vi "Initialize.vi"(8 "error in (no error)":errorcluster, 10 "Device":string) -> (0 "error out":errorcluster, 3 "Force Test Stand out":refnum<class "Force Test Stand.lvclass">)   [LabVIEW 2018, in "Force Test Stand.lvlib" / "Force Test Stand.lvclass"]
uses:
  Force Test Stand.lvclass
  Force Test Stand.lvclass/Force Test Stand.ctl
  builds/Configuration.lvlibp/Configuration.lvclass
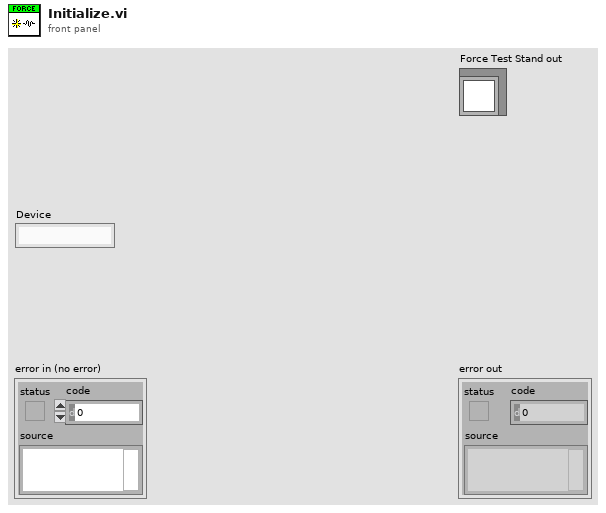
[diagram p1: front panel]
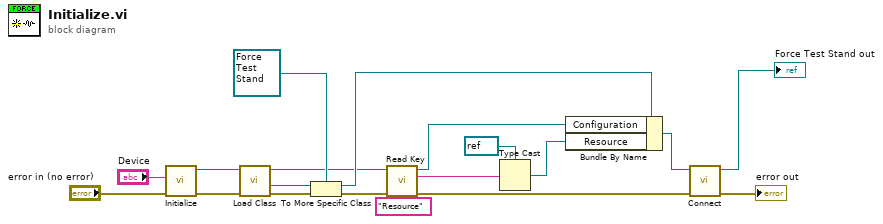
[diagram p0: block diagram]
diagram:
  n1 = call "Initialize.vi"("error in"="error in (no error)", "Device"="Device") -> ("error out"=w16:errorcluster, "Configuration out"=w17:refnum<class "Configuration.lvclass">)  [unwired: 8 in]
  n2 = call "Load Class.vi"("error in"=w16, "Configuration in"=w17) -> ("error out"=w15:errorcluster, "Class out"=w12:refnum<class>, "Configuration out"=w5:refnum<class "Configuration.lvclass">)  [unwired: 7 in]
  n3 = To More Specific Class(target class=refnum<class "Force Test Stand.lvclass"> refnum ("Force Test Stand.lvlib:Force Test Stand.lvclass"), reference=w12, error in=w15) -> (specific class reference=w13:refnum<class "Force Test Stand.lvclass">, error out=w11:errorcluster)
  n4 = call "Read Key.vi"("Key:"="Resource", "error in"=w11, "Configuration in"=w5) -> ("error out"=w10:errorcluster, "Value"=w6:string, "Configuration out"=w3:refnum<class "Configuration.lvclass">)  [unwired: 6 in]
  n5 = Type Cast(type=refnum<visa-resource-name> refnum ("Resource"), x=w6) -> (*(type *) &x=w1:refnum<visa-resource-name>)
  n6 = Bundle By Name(cluster=w13, "Configuration"=w3, "Resource"=w1) -> (w8:refnum<class "Force Test Stand.lvclass">)
  n7 = call-dynamic "Connect.vi"("error in (no error)"=w10, "Force Test Stand in"=w8) -> ("error out"=→"error out":errorcluster, "Force Test Stand out"=→"Force Test Stand out":refnum<class "Force Test Stand.lvclass">)  [unwired: 8 in]
